vi "Check For Existing.vi"(8 "error in (no error)":errorcluster) -> (0 "error out":errorcluster, 2 "Exists?":bool)   [LabVIEW 2013, in "Progress Bar.lvlib"]
uses:
  Progress Bar.lvlib
  Queue/Queue Action.ctl
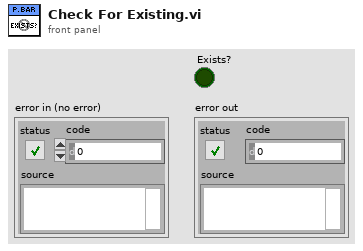
[diagram p1: front panel]
types:
  T1 = typedef "Progress Bar.lvlib/Queue Action.ctl" = enum16{"Obtain Queue", "Release Queue", "Get Queue"}
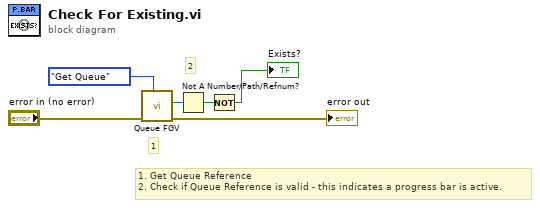
[diagram p0: block diagram]
diagram:
  # "2"
  # "1"
  # "1. Get Queue Reference\n2. Check if Queue Reference is valid - this indicates a progress bar is active."
  n1 = call "Queue FGV.vi"("Enum"=Queue_Action."Get Queue", "error in (no error)"="error in (no error)") -> ("error out"=→"error out":errorcluster, "queue out"=w5:refnum<queue>)  [unwired: 8 in]
  n2 = Not A Number/Path/Refnum?(number/path/refnum=w5) -> (NaN/Path/Refnum?=w2:bool)
  n3 = Not(x=w2) -> (.not. x?=→"Exists?":bool)
